vi "Agilent ReadConfigFile.vi"(7 "Error In":errorcluster) -> (0 "Error Out":errorcluster, 2 "Dispositivos":T1=[["Armario 1", "CH 1", "", ""], ["Armario 1", "CH 2 ", "", ""], ["Armario 1", "CH 3", "", ""], ["Armario 1", "CH 4", "", ""], ["Armario 1", "CH 5", "", ""], ["Armario 1", "CH 6", "", ""], ["Armario 1", "CH 7", "", ""], ["Armario 1", "CH 8", "", ""], ["Armario 2", "CH 1", "", ""], ["Armario 2", "CH 2", "", ""], ["Armario 2", "CH 3", "", ""], ["Armario 2", "CH 4", "", ""], ["Armario 2", "CH 5", "", ""], ["Armario 2", "CH 6", "", ""], ["Armario 2", "CH 7", "", ""], ["Armario 2", "CH 8", "", ""], ["Armario 3", "CH 1", "", ""], ["Armario 3", "CH 2", "", ""], ["Armario 3", "CH 3", "", ""], ["Armario 3", "CH 4", "", ""], ["Armario 3", "CH 5", "", ""], ["Armario 3", "CH 6", "", ""], ["Armario 3", "CH 7", "", ""], ["Armario 3", "CH 8", "", ""], ["Armario 4", "CH 1", "", ""], ["Armario 4", "CH 2", "", ""], ["Armario 4", "CH 3", "", ""], ["Armario 4", "CH 4", "", ""], ["Armario 4", "CH 5", "", ""], ["Armario 4", "CH 6", "", ""], ["Armario 4", "CH 7", "", ""], ["Armario 4", "CH 8", "", ""], ["Armario 5", "CH 1", "", ""], ["Armario 5", "CH 2", "", ""], ["Armario 5", "CH 3", "", ""], ["Armario 5", "CH 4", "", ""], ["Armario 5", "CH 5", "", ""], ["Armario 5", "CH 6", "", ""], ["Armario 5", "CH 7", "", ""], ["Armario 5", "CH 8", "", ""]] caption="configuracionCanales", 3 "configuration file path":path=path "C:/Users/usuario/Documents/LabVIEW Data/canalesAgilentCristalizador.ini")   [LabVIEW 2017]
doc: "Illustrates how to create and write a configuration settings file.\n\nInstructions:\nEnter values in the controls on the front panel then click on the Run Arrow.\nTo read the file, run Read Configuration Settings File.vi located in the file\\config.llb."
uses:
  34970_Configuracion.ctl
  <vilib>/Utility/config.llb/Read Key (String).vi
  <vilib>/Utility/config.llb/NI_LVConfig.lvlib
panel:
  in  "stop":bool
  # "Agilent 34970 informacion\nconfiguración de canales"
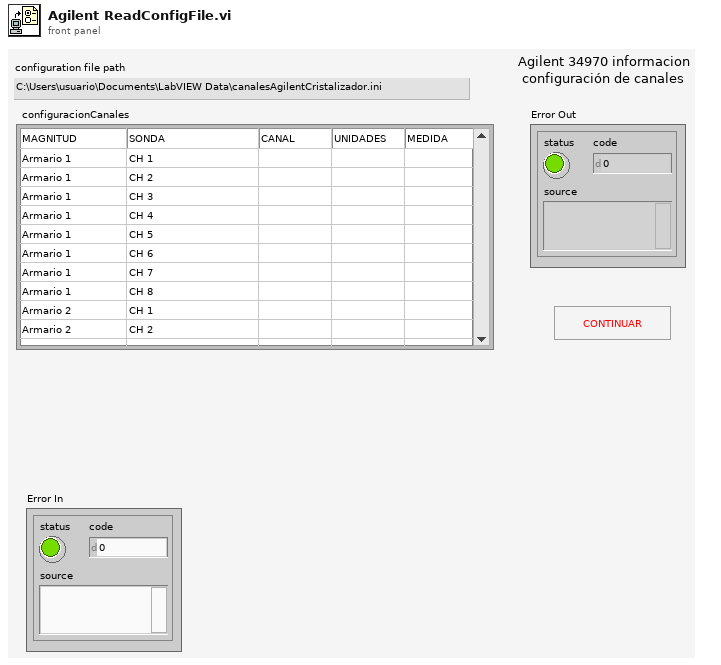
[diagram p1: front panel]
types:
  T1 = typedef "34970_Configuracion.ctl" = string[][]
  T2 = typedef "NI_LVConfig.lvlib/Config Data RefNum.ctl" = refnum<k1>
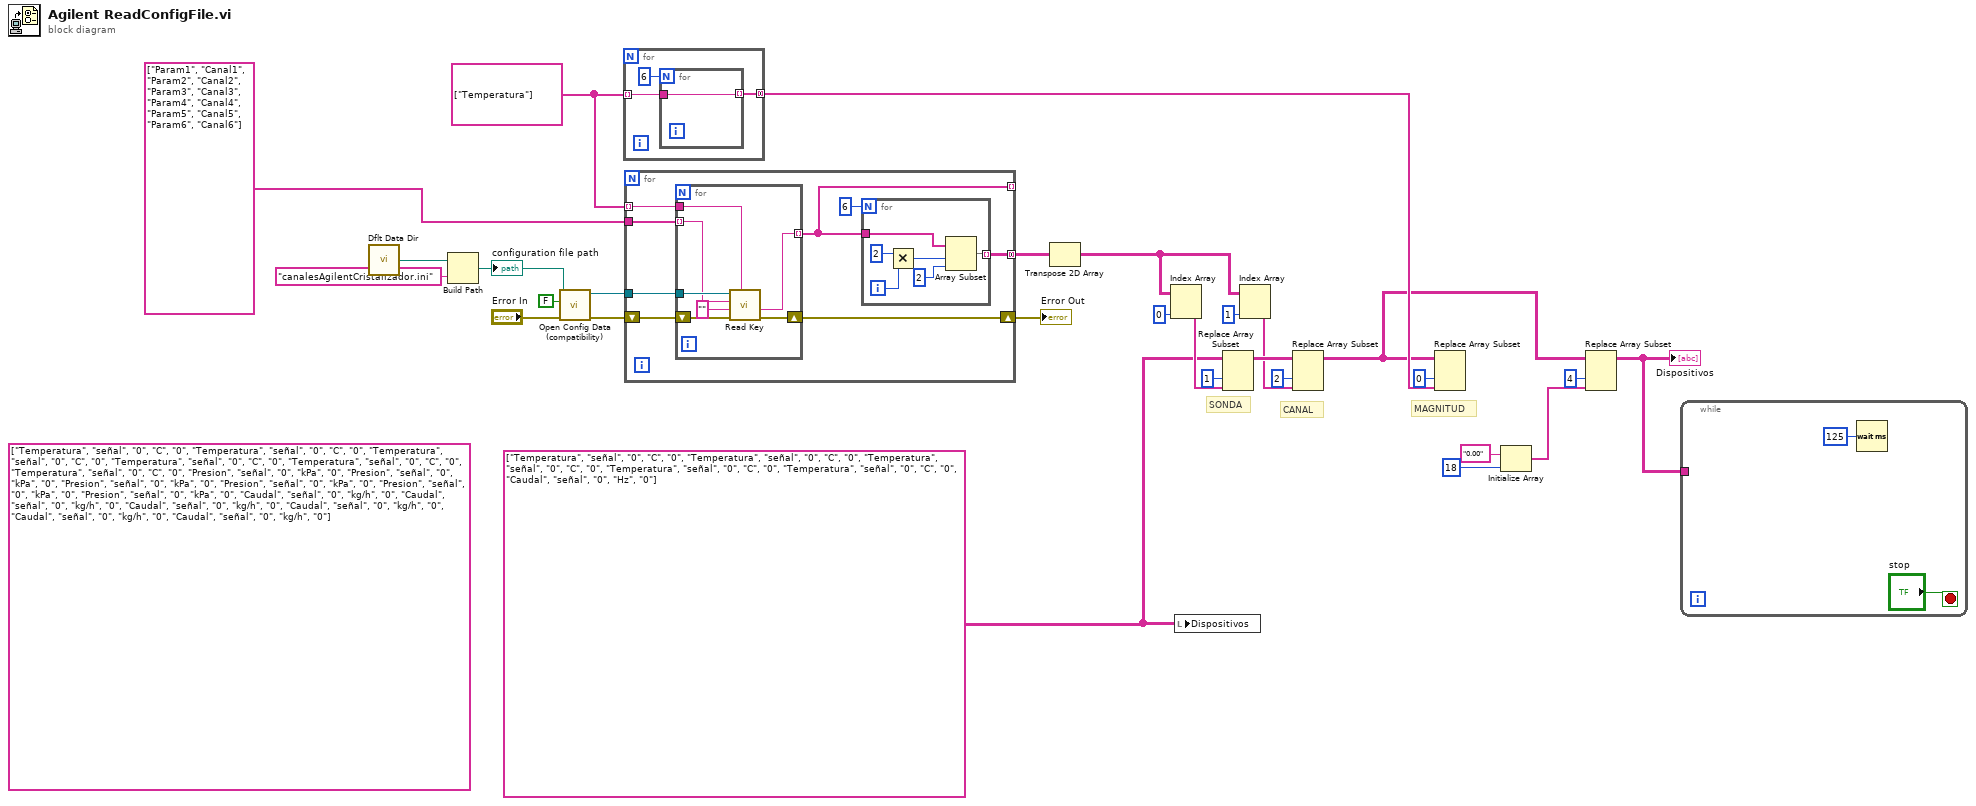
[diagram p0: block diagram]
diagram:
  (unwired) T1 [["Temperatura", "señal", "0", "C", "0"], ["Temperatura", "señal", "0", "C", "0"], ["Temperatura", "señal", "0", "C", "0"], ["Temperatura", "señal", "0", "C", "0"], ["Temperatura", "señal", "0", "C", "0"], ["Temperatura", "señal", "0", "C", "0"], ["Presion", "señal", "0", "kPa", "0"], ["Presion", "señal", "0", "kPa", "0"], ["Presion", "señal", "0", "kPa", "0"], ["Presion", "señal", "0", "kPa", "0"], ["Presion", "señal", "0", "kPa", "0"], ["Presion", "señal", "0", "kPa", "0"], ["Caudal", "señal", "0", "kg/h", "0"], ["Caudal", "señal", "0", "kg/h", "0"], ["Caudal", "señal", "0", "kg/h", "0"], ["Caudal", "señal", "0", "kg/h", "0"], ["Caudal", "señal", "0", "kg/h", "0"], ["Caudal", "señal", "0", "kg/h", "0"]] ("Dispositivos")
  w3 = T1 [["Temperatura", "señal", "0", "C", "0"], ["Temperatura", "señal", "0", "C", "0"], ["Temperatura", "señal", "0", "C", "0"], ["Temperatura", "señal", "0", "C", "0"], ["Temperatura", "señal", "0", "C", "0"], ["Caudal", "señal", "0", "Hz", "0"]] ("Dispositivos")
  w11 = string[] ["Temperatura"]
  # "CANAL"
  # "SONDA"
  # "MAGNITUD"
  n1 = call <vilib>:"Dflt Data Dir.vi"() -> ("App:Default Data Directory"=w26:path)
  n2 = Build Path(base path=w26, name or relative path="canalesAgilentCristalizador.ini") -> (appended path=w4:path)
  "configuration file path" <- w4
  n3 = call <vilib>:"Open Config Data (compatibility).vi"("error in (no error)"="Error In", "create file if necessary (T)"=FALSE ("create file if necessary? (T)"), "configuration file path"=w4) -> ("error out"=w22:errorcluster, "refnum"=w23:T2)  [unwired: 6 in, 1 out]
  n4 = for {
    tunnel: w11 -> [w30] mode=indexing
    tunnel: [w28] -> w9 mode=concatenating
    n5 = for {
      N: 6 -> [_]
      tunnel: w30 -> [w31]
      tunnel: [w31] -> w28 mode=indexing
    }
  }
  n6 = for {
    tunnel: string[] ["Param1", "Canal1", "Param2", "Canal2", "Param3", "Canal3", "Param4", "Canal4", "Param5", "Canal5", "Param6", "Canal6"] -> [w39]
    tunnel: w11 -> [w38] mode=indexing
    tunnel: w23 -> [w37]
    shift-right: [w35] -> w21
    shift-left: w22 -> [w36]
    tunnel: [w33] -> w15 mode=concatenating
    tunnel: [w32] -> _ mode=indexing
    n7 = for {
      tunnel: w38 -> [w46]
      tunnel: w39 -> [w50] mode=indexing
      tunnel: w37 -> [w52]
      shift-right: [w48] -> w35
      shift-left: w36 -> [w51]
      tunnel: [w47] -> w32 mode=indexing
      n8 = call-poly <vilib>:"Read Key.vi"("section"=w46, "error in (no error)"=w51, "default value"="", "key"=w50, "refnum"=w52) -> ("error out"=w48:errorcluster, "value"=w47:string)  [unwired: 3 in, 2 out]
    }
    n9 = for {
      N: 6 -> [_]
      tunnel: w32 -> [w45]
      tunnel: [w40] -> w33 mode=indexing
      i -> [w43]
      n10 = Multiply(x=2 ("index"), y=w43) -> (x*y=w41:i32)
      n11 = Array Subset(array=w45, index=w41, length=2 ("index")) -> (w40:string[])
    }
  }
  "Error Out" <- w21
  n12 = Transpose 2D Array(2D array=w15) -> ()  [unwired: 1 out]
  n13 = Index Array(array=w15, index (col)=0 ("index")) -> (element=w18:string[])  [unwired: 1 in]
  n14 = local write "Dispositivos"(w3) -> ()
  n15 = Replace Array Subset(array=w3, new element=w18, index (col)=1 ("disabled index (col)")) -> (w13:T1)  [unwired: 1 in]
  n16 = Index Array(array=w15, index (col)=1 ("index")) -> (element=w12:string[])  [unwired: 1 in]
  n17 = Replace Array Subset(array=w13, new element=w12, index (col)=2 ("disabled index (col)")) -> (w1:T1)  [unwired: 1 in]
  n18 = Replace Array Subset(array=w1, new element=w9, index (col)=0 ("disabled index (col)")) -> ()  [unwired: 1 in, 1 out]
  n19 = Initialize Array("0.00", 18 ("dimension size")) -> (w5:string[])
  n20 = Replace Array Subset(array=w1, new element=w5, index (col)=4 ("disabled index (col)")) -> (w2:T1)  [unwired: 1 in]
  "Dispositivos" <- w2
  n21 = while {
    tunnel: w2 -> [_]
    stop <- "stop" stop-if-true
    n22 = Wait (ms)(milliseconds to wait=u32 125) -> ()  [unwired: 1 out]
  }
